vi "Sys Config-format and values.vi"(0 "System Config":T4={"XY Stage"={"COM port"="", "XY stage available"=FALSE, "Baudrate"=0, "Type"=""}, "DAQ FPGA"={"Target"="RIO0", "input card type"=enum."AC Card", "Ref"=refnum, "Clock Freq (MHz) "=200.0, "Samples Wait after Trigger"=5080, "AOD fill"=4900, "StartupDelay"=0, "Slip Cycle (clock cycles)"=600000, "Add Cycle"=TRUE}, "Control system"={"Contrl Sys Available Ind"=FALSE, "Control system.FPGA Type"=enum."Virtex 5", "Control system.Network adapter name"="", "Control system.MAC address"="", "Control system.Ethernet Port"=0, "Ethernet opened"=FALSE, "Ctrl FPGA Clock (MHz)"=240.0, "AOD 1 Amplitude"=0, "AOD 2 Amplitude"=0, "AOD 3 Amplitude"=0, "AOD 4 Amplitude"=0, "AOD 5 Amplitude"=0, "AOD 6 Amplitude"=0, "Data Time Interval (ns)"=0.0, "T0 (ns)"=0.0, "Ta (ns)"=0.0}, "Encoder"={"IP address"="224.0.1.103", "Port"=7000, "Wheel radius (cm)"=16.0, "Encoder Trigger"=""}, "DAQmx Chan"={"Pockels AO"="", "Hard shutter AO"="", "PMT AOs"="", "Galvo AOs"="", "Power meter AI"=""}, "Computer MAC address"="", "Cam VidRec"={"DO flag-Video record"="", "DO flag-Trial start"=""}, "Externalise Triggers"=FALSE, "MC Supported"=FALSE, "Laser wavelength (nm)"=920.0} {"Laser wavelength (nm)" min=800.0 max=1080.0 step=1.0; "Encoder"."Wheel radius (cm)" format="%#_13g"; "Control system"."Control system.Ethernet Port" min=0 max=2048 step=1; "Control system"."Ctrl FPGA Clock (MHz)" min=80.0 max=500.0 step=1.0; "Control system"."Data Time Interval (ns)" min=0.0 max=2048.0 step=1.0; "Control system"."Ta (ns)" min=0.0 max=2048.0 step=1.0; "Control system"."T0 (ns)" min=0.0 max=2048.0 step=1.0; "Control system"."AOD 6 Amplitude" min=0 max=2048 step=1; "Control system"."AOD 5 Amplitude" min=0 max=2048 step=1; "Control system"."AOD 4 Amplitude" min=0 max=2048 step=1; "Control system"."AOD 3 Amplitude" min=0 max=2048 step=1; "Control system"."AOD 2 Amplitude" min=0 max=2048 step=1; "Control system"."AOD 1 Amplitude" min=0 max=2048 step=1}) -> (13 "error out":errorcluster, 14 "Keys setup.DBL":T2=[{"key"="Control FPGA.Clock Freq (MHz)", "Save?"=TRUE, "Default"=240.0}, {"key"="DAQ FPGA.Clock Freq (MHz)", "Save?"=TRUE, "Default"=240.0}], 15 "Values.DBL":dbl[](array[numeric]), 16 "Keys setup.String":T3=[{"key"="Control FPGA.MAC address", "Save?"=TRUE, "Default"="AABBCCDDEEFF"}, {"key"="DAQ FPGA.Target", "Save?"=TRUE, "Default"="RIO0"}, {"key"="XY Stage.COM port", "Save?"=TRUE, "Default"="COM7"}, {"key"="DAQmx Chan.Pockels Control", "Save?"=TRUE, "Default"=""}, {"key"="DAQmx Chan.Hard Shutter", "Save?"=TRUE, "Default"=""}, {"key"="DAQmx Chan.PMT 1", "Save?"=TRUE, "Default"=""}, {"key"="DAQmx Chan.PMT 2", "Save?"=TRUE, "Default"=""}, {"key"="DAQmx Chan.Encoder Trigger", "Save?"=TRUE, "Default"=""}, {"key"="DAQmx Chan.Optional Trigger 1", "Save?"=TRUE, "Default"=""}, {"key"="DAQmx Chan.Optional Trigger 2", "Save?"=TRUE, "Default"=""}, {"key"="DAQmx Chan.Optional Trigger 3", "Save?"=TRUE, "Default"=""}], 17 "Values.Strings":string[](array[string]), 18 "Keys setup.Boolean":T1, 19 "Values.Boolean":bool[](array[boolean]))   [LabVIEW 2017]
uses:
  Typedefs/Ini file interface (DBL).ctl
  Typedefs/Ini file interface (String).ctl
  Typedefs/Ini file interface (Boolean).ctl
  Typedefs/XY Stage config cluster.ctl
  <vilib>/userdefined/High Color/nirio_resource_hc.ctl
  RIG-SPECIFIC FILES/FPGA Refs/FPGA Ref.ctl
  Typedefs/DAQ FPGA config cluster.ctl
  Typedefs/DAQmx physical channels cluster.ctl
  Typedefs/CTRL system config cluster.ctl
  Typedefs/Sys Configuration.ctl
  Typedefs/FPGA input type AC-DC.ctl
  Typedefs/Encoder config cluster.ctl
  Typedefs/Cam VidRec HW config setup cluster.ctl
panel:
  # "NOTES:\n1. \"Control FPGA.Ethernet port\" is detected automatically. It is not saved/loaded from file.\n2. \"Control FPGA.Ethernet Opened\" is detected automatically. It is not saved/loaded from file."
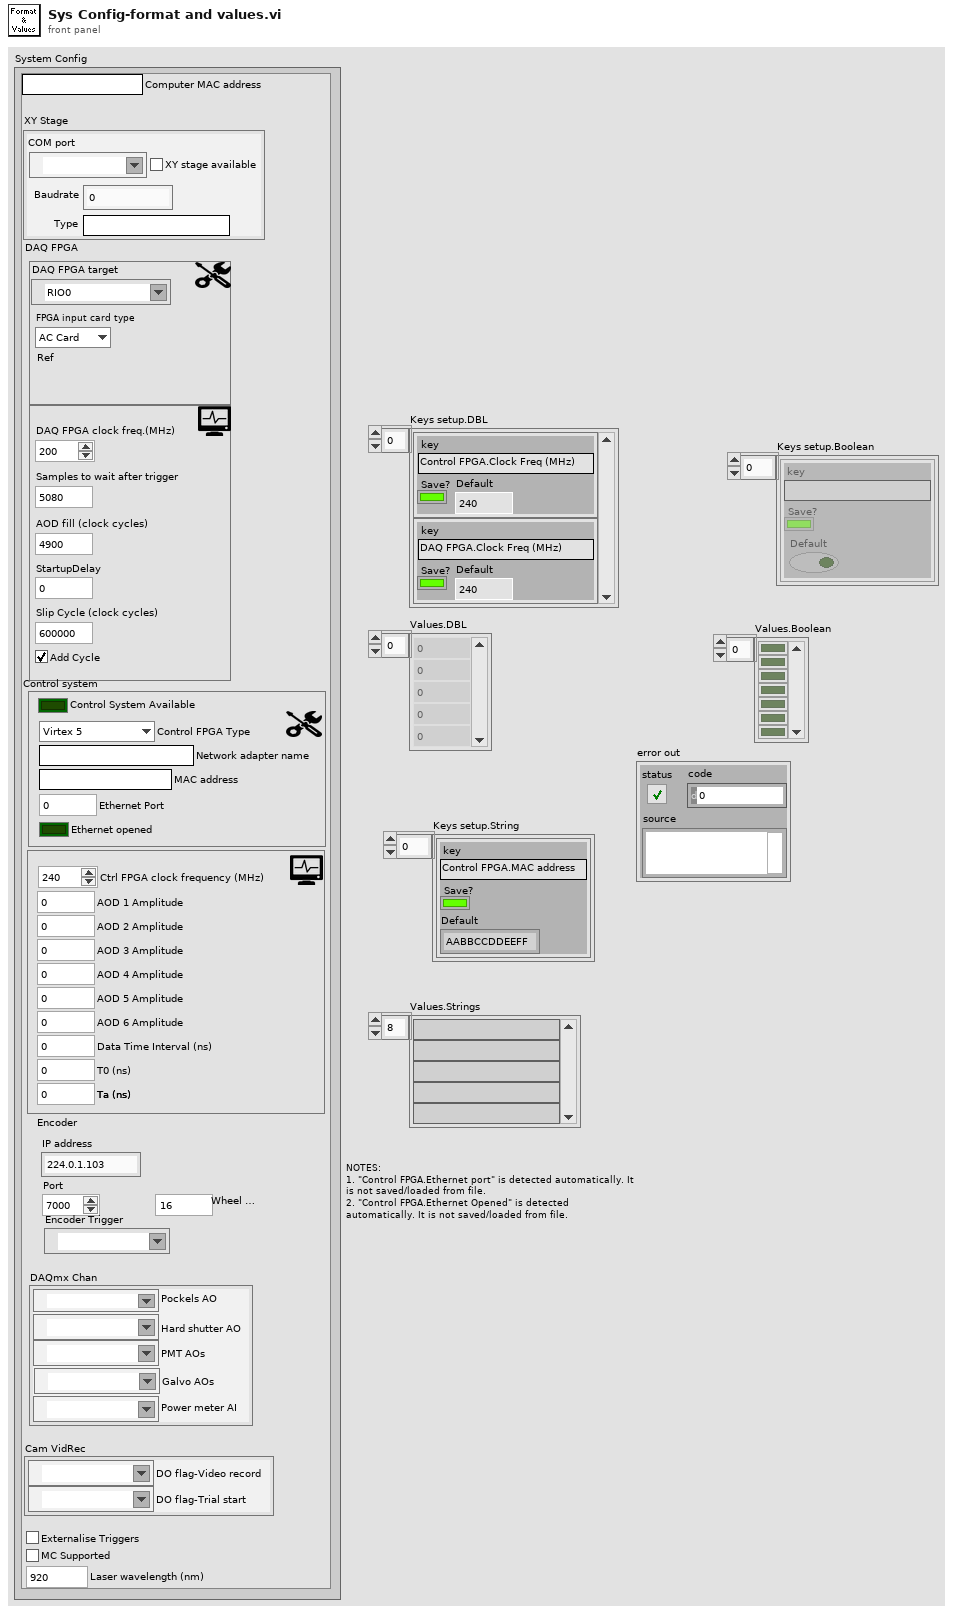
[diagram p1: front panel]
types:
  T1 = typedef "Ini file interface (Boolean).ctl" = cluster{"key":string, "Save?":bool, "Default":bool}[]
  T2 = typedef "Ini file interface (DBL).ctl" = cluster{"key":string, "Save?":bool, "Default":dbl}[]
  T3 = typedef "Ini file interface (String).ctl" = cluster{"key":string, "Save?":bool, "Default":string}[]
  T4 = typedef "Sys Configuration.ctl" = cluster{"XY Stage":T5, "DAQ FPGA":T6, "Control system":T10, "Encoder":T11, "DAQmx Chan":T12, "Computer MAC address":string, "Cam VidRec":T13, "Externalise Triggers":bool, "MC Supported":bool, "Laser wavelength (nm)":dbl}
  T5 = typedef "XY Stage config cluster.ctl" = cluster{"COM port":refnum<visa-resource-name>, "XY stage available":bool, "Baudrate":i32, "Type":string}
  T6 = typedef "DAQ FPGA config cluster.ctl" = cluster{"Target":T7, "input card type":T8, "Ref":T9, "Clock Freq (MHz) ":dbl, "Samples Wait after Trigger":u16, "AOD fill":u16, "StartupDelay":i32, "Slip Cycle (clock cycles)":u32, "Add Cycle":bool}
  T7 = typedef "nirio_resource_hc.ctl" = tag
  T8 = typedef "FPGA input type AC-DC.ctl" = enum16{"AC Card", "DC Card"}
  T9 = typedef "FPGA Ref.ctl" = refnum<k20>
  T10 = typedef "CTRL system config cluster.ctl" = cluster{"Contrl Sys Available Ind":bool, "Control system.FPGA Type":enum16{"Virtex 5", "Virtex 7"}, "Control system.Network adapter name":string, "Control system.MAC address":string, "Control system.Ethernet Port":i16, "Ethernet opened":bool, "Ctrl FPGA Clock (MHz)":dbl, "AOD 1 Amplitude":i16, "AOD 2 Amplitude":i16, "AOD 3 Amplitude":i16, "AOD 4 Amplitude":i16, "AOD 5 Amplitude":i16, "AOD 6 Amplitude":i16, "Data Time Interval (ns)":dbl, "T0 (ns)":dbl, "Ta (ns)":dbl}
  T11 = typedef "Encoder config cluster.ctl" = cluster{"IP address":string, "Port":u16, "Wheel radius (cm)":dbl, "Encoder Trigger":tag}
  T12 = typedef "DAQmx physical channels cluster.ctl" = cluster{"Pockels AO":tag, "Hard shutter AO":tag, "PMT AOs":tag, "Galvo AOs":tag, "Power meter AI":tag}
  T13 = typedef "Cam VidRec HW config setup cluster.ctl" = cluster{"DO flag-Video record":tag, "DO flag-Trial start":tag}
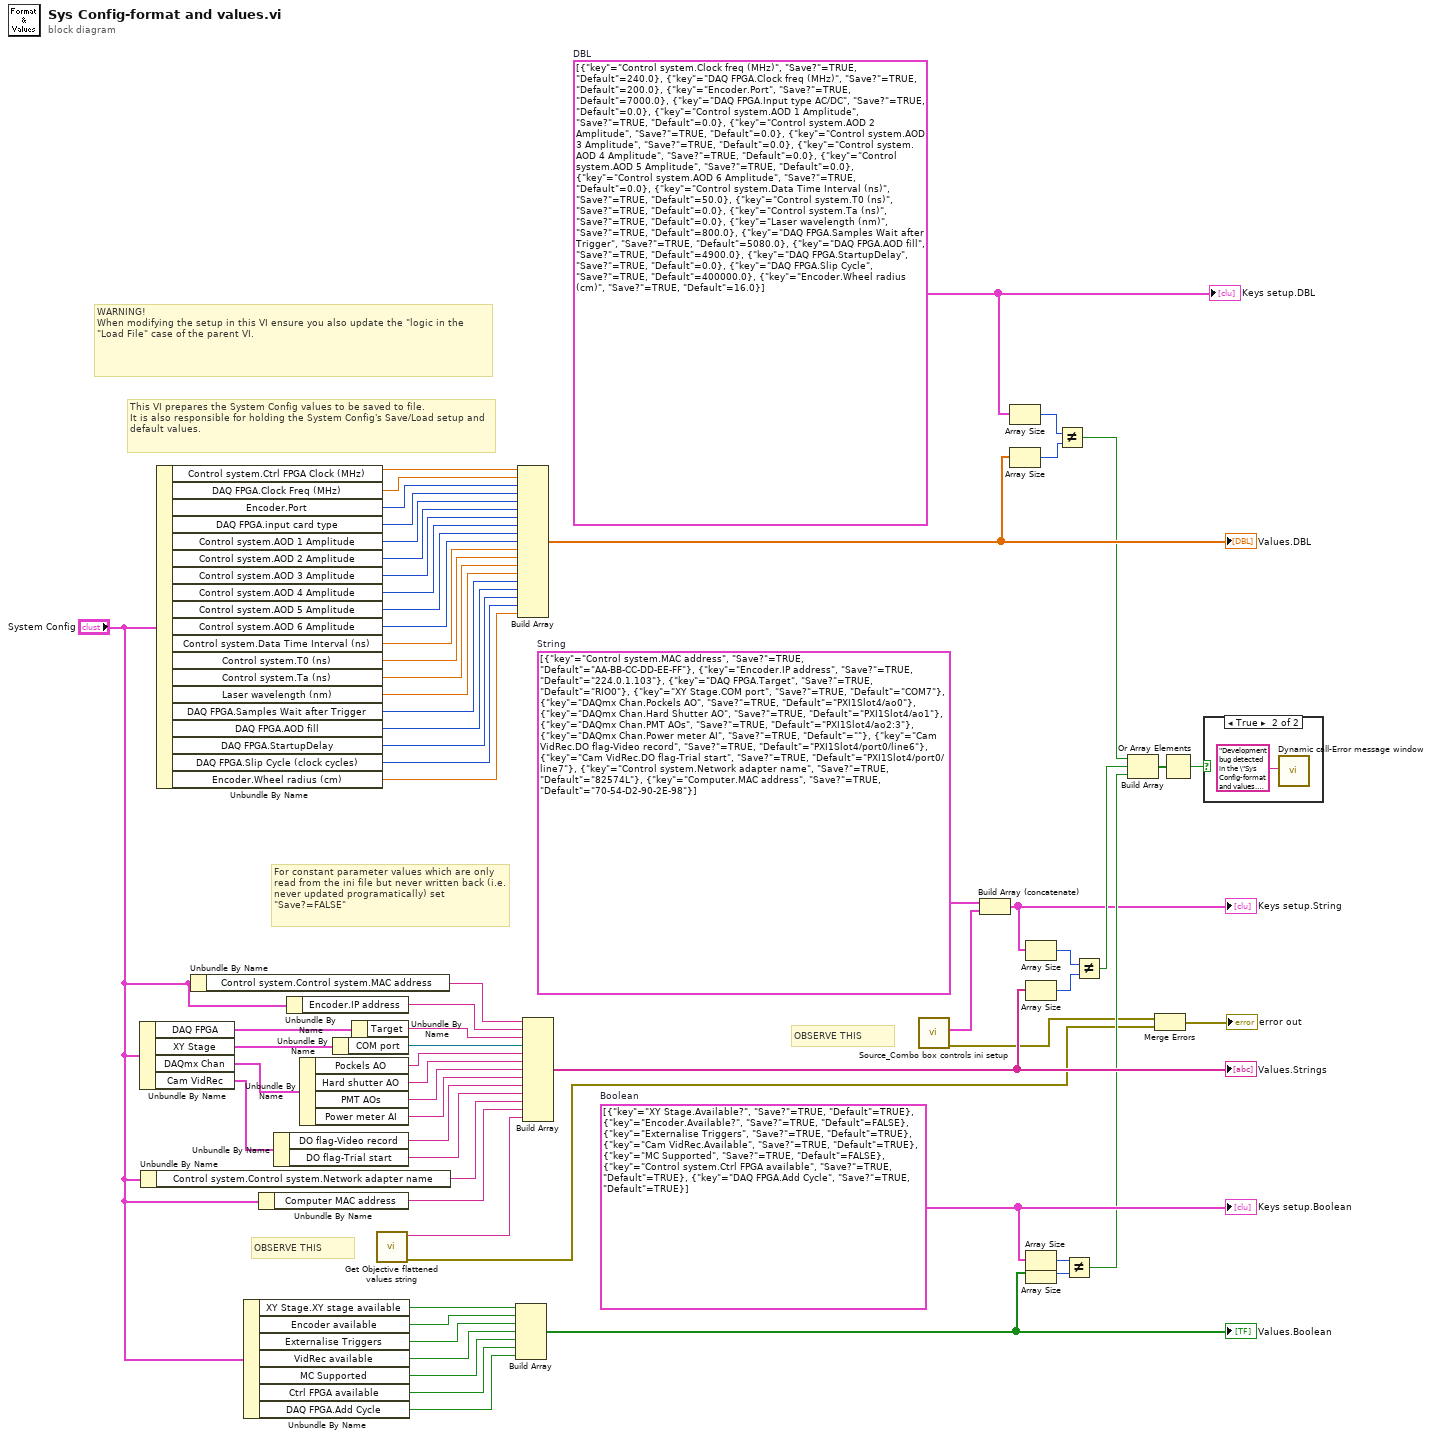
[diagram p0: block diagram]
diagram:
  w54 = T1 [{"key"="XY Stage.Available?", "Save?"=TRUE, "Default"=TRUE}, {"key"="Encoder.Available?", "Save?"=TRUE, "Default"=FALSE}, {"key"="Externalise Triggers", "Save?"=TRUE, "Default"=TRUE}, {"key"="Cam VidRec.Available", "Save?"=TRUE, "Default"=TRUE}, {"key"="MC Supported", "Save?"=TRUE, "Default"=FALSE}, {"key"="Control system.Ctrl FPGA available", "Save?"=TRUE, "Default"=TRUE}, {"key"="DAQ FPGA.Add Cycle", "Save?"=TRUE, "Default"=TRUE}]  # Boolean
  w9 = T3 [{"key"="Control system.MAC address", "Save?"=TRUE, "Default"="AA-BB-CC-DD-EE-FF"}, {"key"="Encoder.IP address", "Save?"=TRUE, "Default"="224.0.1.103"}, {"key"="DAQ FPGA.Target", "Save?"=TRUE, "Default"="RIO0"}, {"key"="XY Stage.COM port", "Save?"=TRUE, "Default"="COM7"}, {"key"="DAQmx Chan.Pockels AO", "Save?"=TRUE, "Default"="PXI1Slot4/ao0"}, {"key"="DAQmx Chan.Hard Shutter AO", "Save?"=TRUE, "Default"="PXI1Slot4/ao1"}, {"key"="DAQmx Chan.PMT AOs", "Save?"=TRUE, "Default"="PXI1Slot4/ao2:3"}, {"key"="DAQmx Chan.Power meter AI", "Save?"=TRUE, "Default"=""}, {"key"="Cam VidRec.DO flag-Video record", "Save?"=TRUE, "Default"="PXI1Slot4/port0/line6"}, {"key"="Cam VidRec.DO flag-Trial start", "Save?"=TRUE, "Default"="PXI1Slot4/port0/line7"}, {"key"="Control system.Network adapter name", "Save?"=TRUE, "Default"="82574L"}, {"key"="Computer.MAC address", "Save?"=TRUE, "Default"="70-54-D2-90-2E-98"}]  # String
  w57 = T2 [{"key"="Control system.Clock freq (MHz)", "Save?"=TRUE, "Default"=240.0}, {"key"="DAQ FPGA.Clock freq (MHz)", "Save?"=TRUE, "Default"=200.0}, {"key"="Encoder.Port", "Save?"=TRUE, "Default"=7000.0}, {"key"="DAQ FPGA.Input type AC/DC", "Save?"=TRUE, "Default"=0.0}, {"key"="Control system.AOD 1 Amplitude", "Save?"=TRUE, "Default"=0.0}, {"key"="Control system.AOD 2 Amplitude", "Save?"=TRUE, "Default"=0.0}, {"key"="Control system.AOD 3 Amplitude", "Save?"=TRUE, "Default"=0.0}, {"key"="Control system.AOD 4 Amplitude", "Save?"=TRUE, "Default"=0.0}, {"key"="Control system.AOD 5 Amplitude", "Save?"=TRUE, "Default"=0.0}, {"key"="Control system.AOD 6 Amplitude", "Save?"=TRUE, "Default"=0.0}, {"key"="Control system.Data Time Interval (ns)", "Save?"=TRUE, "Default"=50.0}, {"key"="Control system.T0 (ns)", "Save?"=TRUE, "Default"=0.0}, {"key"="Control system.Ta (ns)", "Save?"=TRUE, "Default"=0.0}, {"key"="Laser wavelength (nm)", "Save?"=TRUE, "Default"=800.0}, {"key"="DAQ FPGA.Samples Wait after Trigger", "Save?"=TRUE, "Default"=5080.0}, {"key"="DAQ FPGA.AOD fill", "Save?"=TRUE, "Default"=4900.0}, {"key"="DAQ FPGA.StartupDelay", "Save?"=TRUE, "Default"=0.0}, {"key"="DAQ FPGA.Slip Cycle", "Save?"=TRUE, "Default"=400000.0}, {"key"="Encoder.Wheel radius (cm)", "Save?"=TRUE, "Default"=16.0}]  # DBL
  # "OBSERVE THIS"
  # "OBSERVE THIS"
  # "WARNING!\nWhen modifying the setup in this VI ensure you also update the \"logic in the \"Load File\" case of the parent VI."
  # "For constant parameter values which are only read from the ini file but never written back (i.e. never updated programatically) set \"Save?=FALSE\""
  # "This VI prepares the System Config values to be saved to file.\nIt is also responsible for holding the System Config's Save/Load setup and default values."
  n1 = Unbundle By Name("System Config") -> ("DAQ FPGA"=w61:T6, "XY Stage"=w63:T5, "DAQmx Chan"=w66:T12, "Cam VidRec"=w27:T13)
  n2 = Unbundle By Name("System Config") -> ("Control system.Control system.Network adapter name"=w37:string)
  n3 = Unbundle By Name("System Config") -> ("Control system.Ctrl FPGA Clock (MHz)"=w58:dbl, "DAQ FPGA.Clock Freq (MHz)"=w40:dbl, "Encoder.Port"=w39:u16, "DAQ FPGA.input card type"=w38:T8, "Control system.AOD 1 Amplitude"=w25:i16, "Control system.AOD 2 Amplitude"=w24:i16, "Control system.AOD 3 Amplitude"=w23:i16, "Control system.AOD 4 Amplitude"=w22:i16, "Control system.AOD 5 Amplitude"=w21:i16, "Control system.AOD 6 Amplitude"=w20:i16, "Control system.Data Time Interval (ns)"=w18:dbl, "Control system.T0 (ns)"=w17:dbl, "Control system.Ta (ns)"=w16:dbl, "Laser wavelength (nm)"=w15:dbl, "DAQ FPGA.Samples Wait after Trigger"=w14:u16, "DAQ FPGA.AOD fill"=w13:u16, "DAQ FPGA.StartupDelay"=w12:i32, "DAQ FPGA.Slip Cycle (clock cycles)"=w11:u32, "Encoder.Wheel radius (cm)"=w4:dbl)
  n4 = Unbundle By Name("System Config") -> ("Control system.Control system.MAC address"=w42:string)
  n5 = Unbundle By Name("System Config") -> ("XY Stage.XY stage available"=w34:bool, "Encoder available"=w35:bool, "Externalise Triggers"=w31:bool, "VidRec available"=w30:bool, "MC Supported"=w26:bool, "Ctrl FPGA available"=w19:bool, "DAQ FPGA.Add Cycle"=w10:bool)
  n6 = Unbundle By Name("System Config") -> ("Computer MAC address"=w36:string)
  n7 = Unbundle By Name(w27) -> ("DO flag-Video record"=w29:tag, "DO flag-Trial start"=w28:tag)
  n8 = Unbundle By Name("System Config") -> ("Encoder.IP address"=w41:string)
  n9 = Unbundle By Name(w66) -> ("Pockels AO"=w62:tag, "Hard shutter AO"=w65:tag, "PMT AOs"=w64:tag, "Power meter AI"=w5:tag)
  n10 = Unbundle By Name(w63) -> ("COM port"=w60:refnum<visa-resource-name>)
  n11 = Unbundle By Name(w61) -> ("Target"=w59:T7)
  n12 = call "Get Objective flattened values string.vi"() -> ("error out"=w2:errorcluster, "\"Objective\" control's flattened values string"=w6:string)  [unwired: 9 in, 1 out]
  n13 = Build Array(w34, w35, w31, w30, w26, w19, w10) -> (w32:bool[])
  "Values.Boolean" <- w32
  n14 = Build Array(w58, w40, w39, w38, w25, w24, w23, w22, w21, w20, w18, w17, w16, w15, w14, w13, w12, w11, w4) -> (w55:dbl[])
  "Values.DBL" <- w55
  n15 = Build Array(w42, w41, w59, w60, w62, w65, w64, w5, w29, w28, w37, w36, w6) -> (w56:string[])
  "Values.Strings" <- w56
  n16 = call "Source_Combo box controls ini setup.vi"() -> ("error out"=w3:errorcluster, "Keys setup"=w7:T3)  [unwired: 9 in, 1 out]
  n17 = Build Array (concatenate)(w9, w7) -> (w8:T3)
  "Keys setup.String" <- w8
  n18 = Array Size(array=w57) -> (size(s)=w51:i32)
  n19 = Array Size(array=w55) -> (size(s)=w50:i32)
  n20 = Array Size(array=w8) -> (size(s)=w53:i32)
  n21 = Array Size(array=w56) -> (size(s)=w52:i32)
  n22 = Array Size(array=w54) -> (size(s)=w49:i32)
  n23 = Array Size(array=w32) -> (size(s)=w48:i32)
  n24 = Not Equal?(x=w51, y=w50) -> (x != y?=w44:bool)
  n25 = Not Equal?(x=w49, y=w48) -> (x != y?=w46:bool)
  n26 = Not Equal?(x=w53, y=w52) -> (x != y?=w43:bool)
  n27 = Build Array(w44, w43, w46) -> (w47:bool[])
  n28 = Merge Errors(w3, w2) -> (→"error out":errorcluster)
  n29 = Or Array Elements(Boolean array=w47) -> (logical OR=w45:bool)
  n30 = case shown="True" w45 {
    frame False {
    }
    frame True {
      n31 = call "Dynamic call-Error message window.vi"("Error Message"="Development bug detected in the \"Sys Config-format and values.vi\".\nPlease correct the set up in this VI.") -> ()  [unwired: 10 in, 1 out]
    }
  }
  "Keys setup.DBL" <- w57
  "Keys setup.Boolean" <- w54
